vi "Control Panel.vi"(8 "error in (no error)":errorcluster, 11 "Power Supply.lvclass":refnum<class "Power Supply.lvclass">) -> (0 "error out":errorcluster, 3 "Power Supply.lvclass out":refnum<class "Power Supply.lvclass">)   [LabVIEW 2009, in "Power Supply.lvclass"]
uses:
  Power Supply.lvclass
  Utility Classes/InstrPtr/InstrPtr.lvclass
  Magnet status.ctl
  Power Supply.lvclass/Power Supply.ctl
  Global/Relative Sound Files.vi
  File IO/File IO.lvclass
panel:
  out "Was at persistent?":bool
  in  "Return to \npersistent?":bool
  out "log counter":dbl
  out "Going to Field?":bool
  out "Current Field":dbl[unit]
  out "Update UI":bool
  out "Status":T1
  out "*ips120":T2
  in  "Abort Field Sweep":bool
  out "done?":bool
  out "ILM Shut Down?":bool
  out "SH On":bool caption="Switch Heater"
  out "Persistent Mode":bool
  in  "SHcontrol":bool caption="Switch Heater"
  in  "gotopersistent":bool
  out "active":bool
  in  "Train\nMagnet":bool
  out "Busy":bool
  out "ready?":bool
  in  "rate":dbl[unit]=0.016666666666666666 caption="Rate" min=0.0 max=0.25
  in  "Goto":dbl[unit]
  in  "Clamp":bool
  in  "Check for Magnet":bool
  in  "Hold":bool
  in  "Goto Zero":bool
  in  "Goto Field":bool
  in  "endprgm":bool
  # "Magnet Control Panel"
  # "(at current field)"
  # "Off"
  # "On"
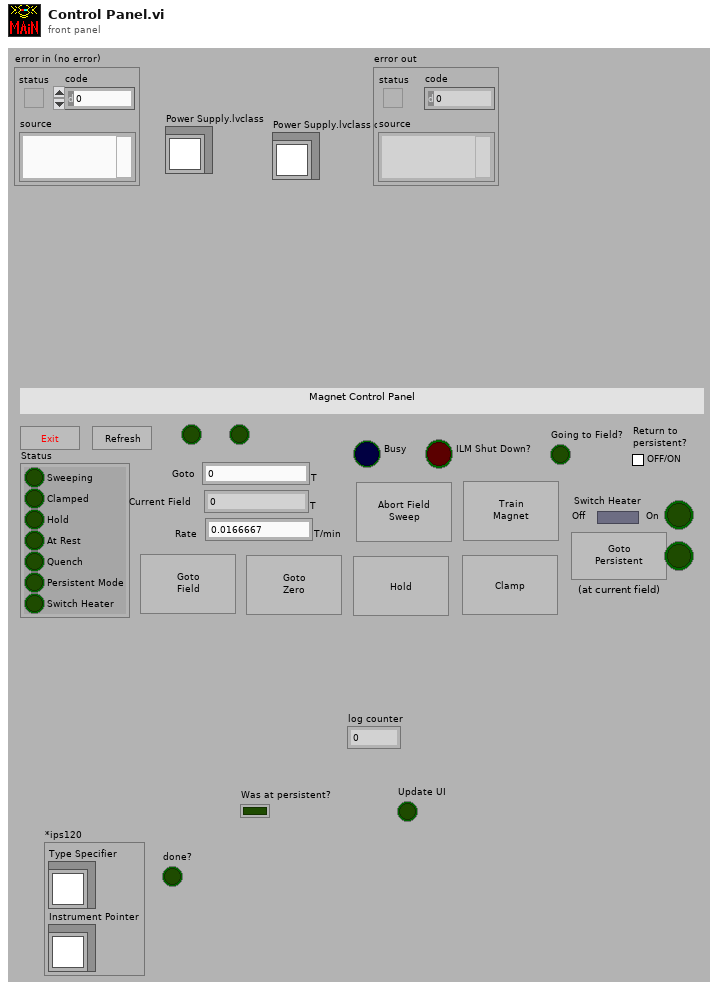
[diagram p1: front panel]
types:
  T1 = typedef "Power Supply.lvclass/Magnet status.ctl" = cluster{"Sweeping":bool, "Clamped":bool, "Hold":bool, "At Rest":bool, "Quench":bool, "Persistent Mode":bool, "Switch Heater":bool}
  T2 = cluster{"Type Specifier":refnum<class "Power Supply.lvclass">, "Instrument Pointer":refnum<class "InstrPtr.lvclass">}
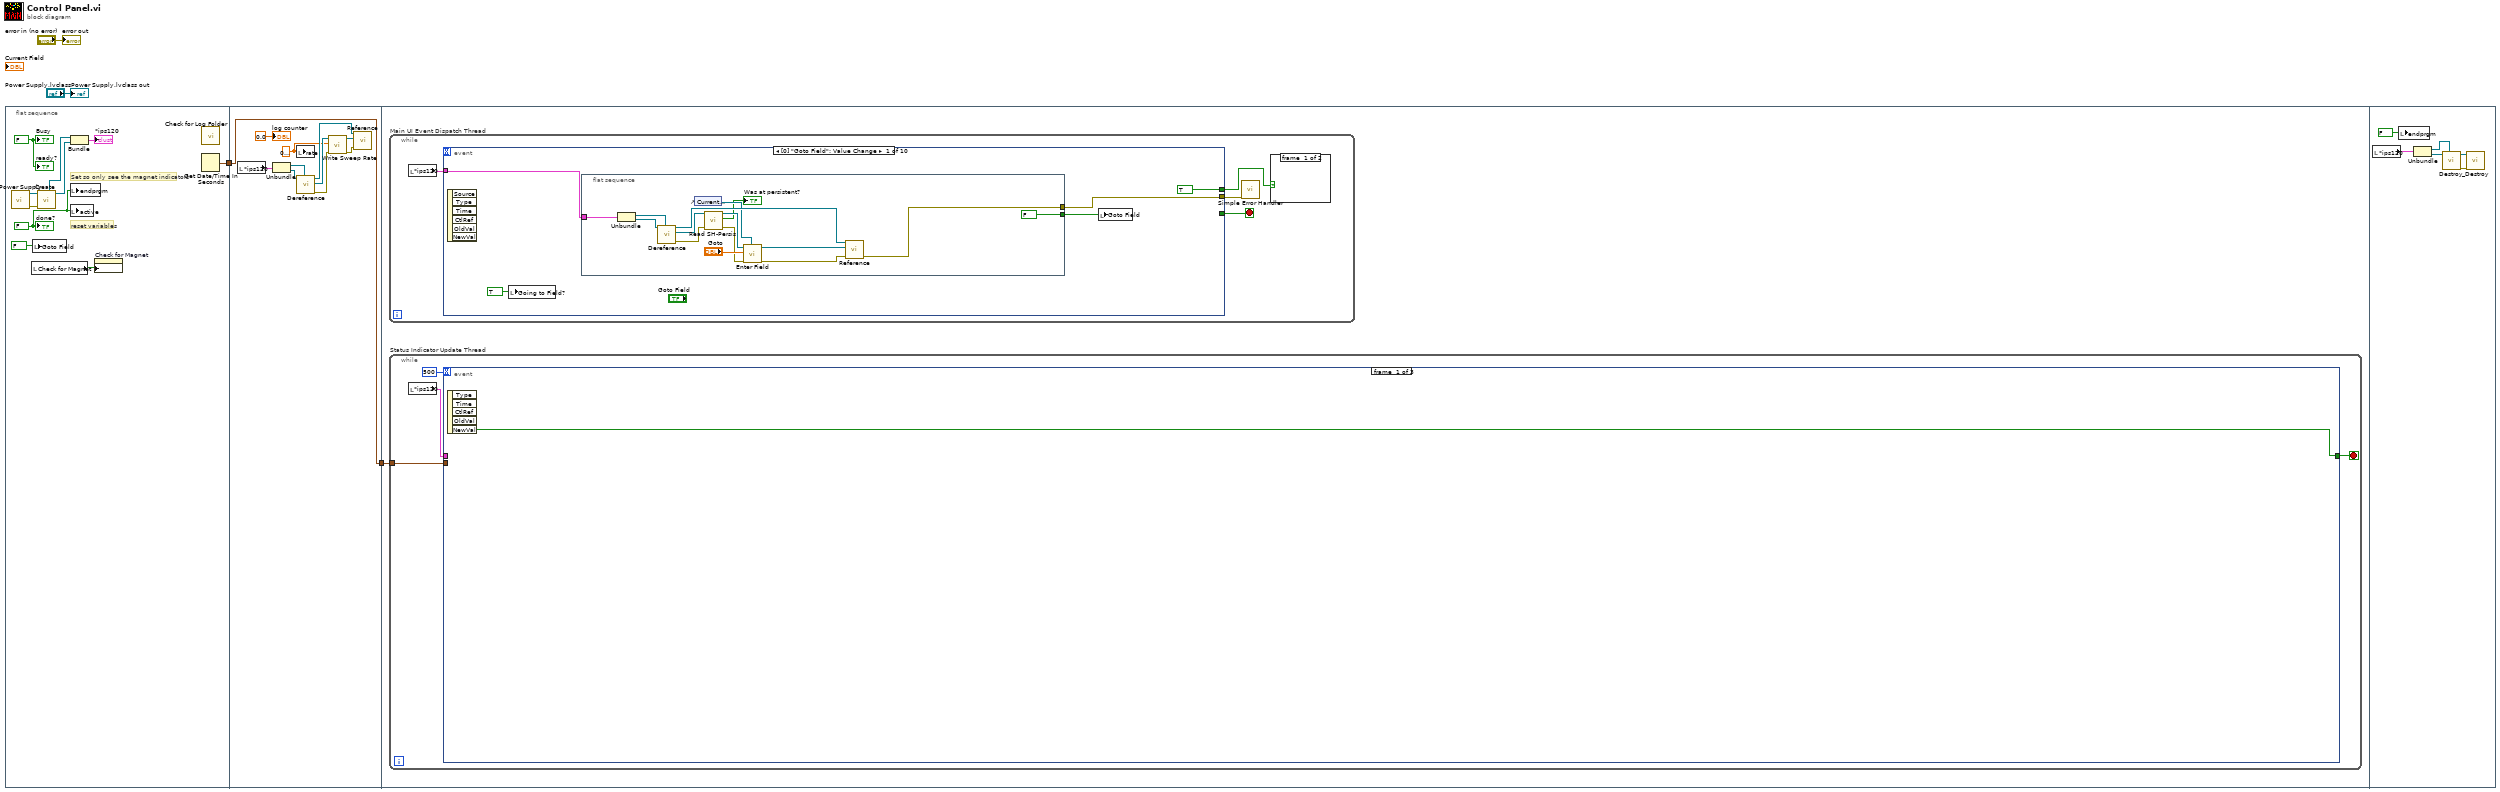
[diagram p0: block diagram]
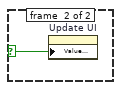
[diagram p2: hidden frame]
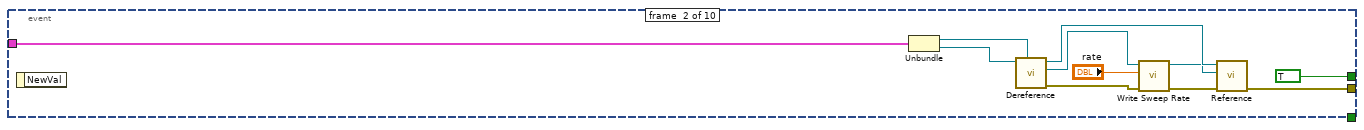
[diagram p3: hidden frame]
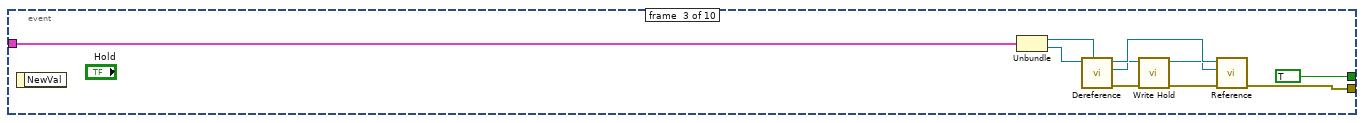
[diagram p4: hidden frame]
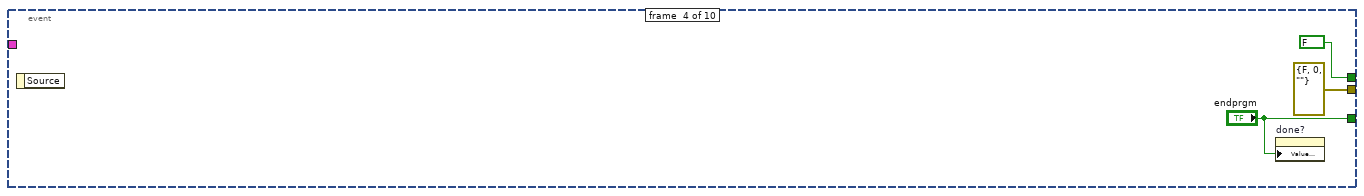
[diagram p5: hidden frame]
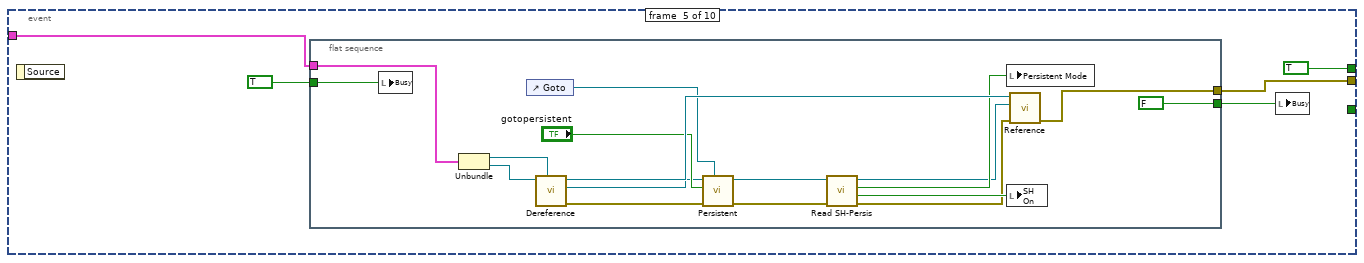
[diagram p6: hidden frame]
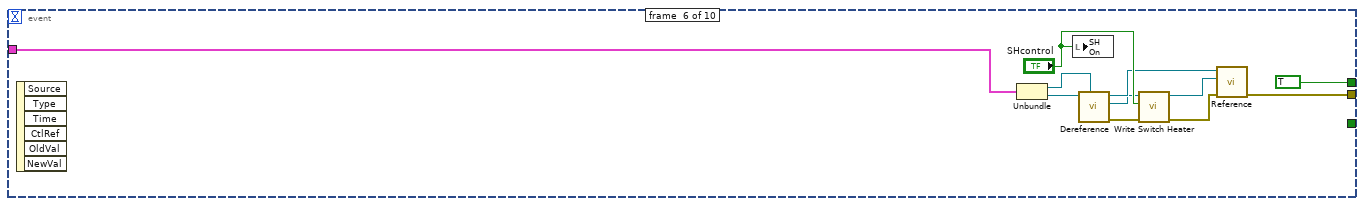
[diagram p7: hidden frame]
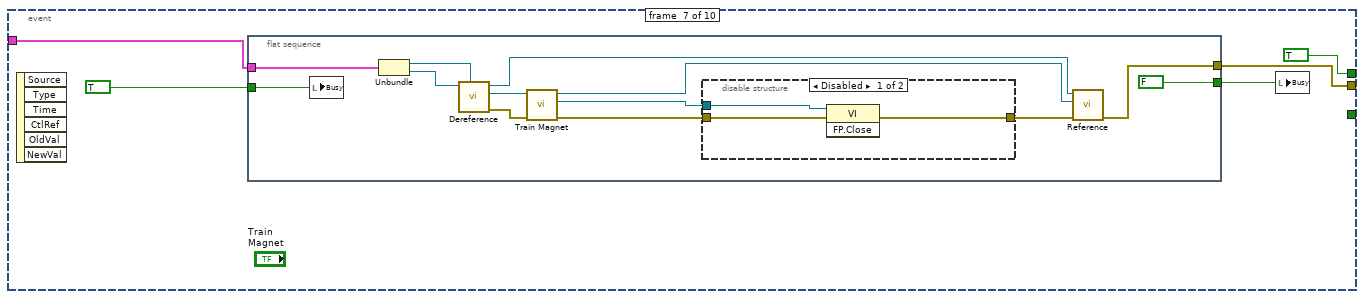
[diagram p8: hidden frame]
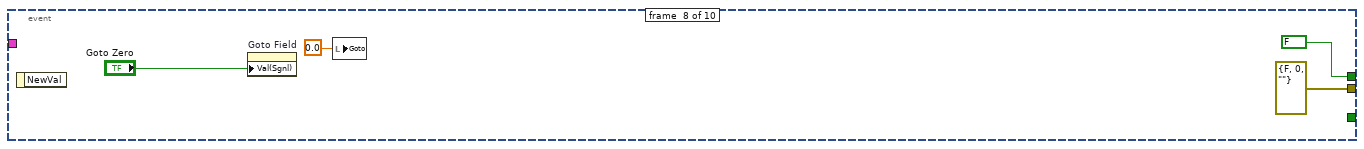
[diagram p10: hidden frame]
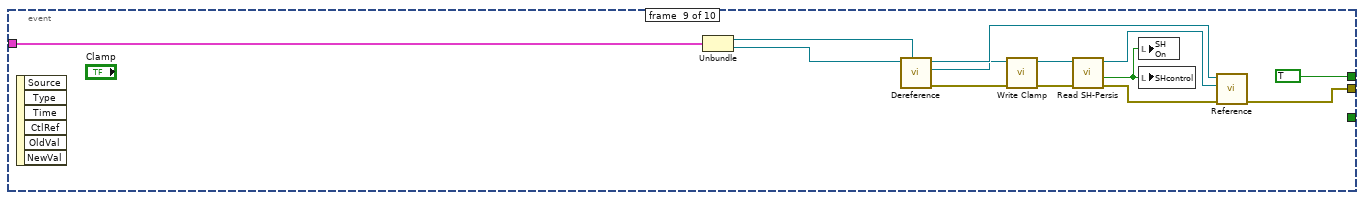
[diagram p11: hidden frame]
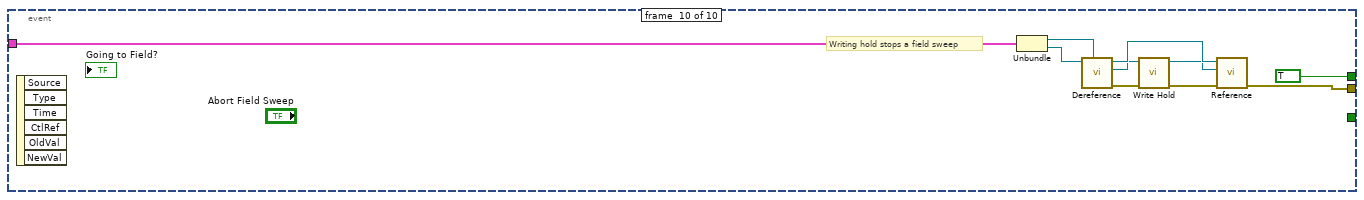
[diagram p12: hidden frame]
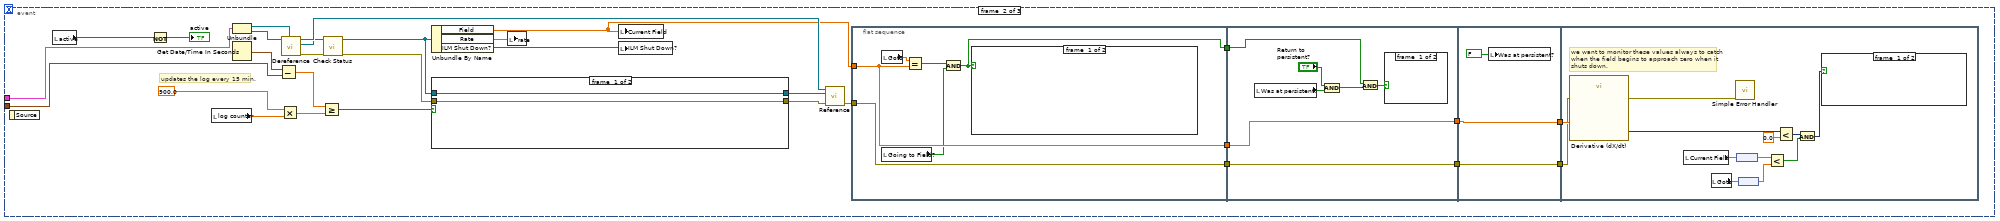
[diagram p13: hidden frame]
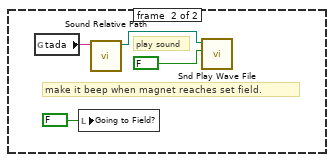
[diagram p14: hidden frame]
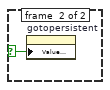
[diagram p15: hidden frame]
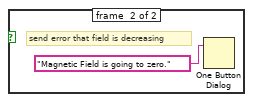
[diagram p16: hidden frame]
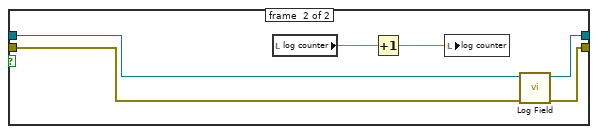
[diagram p17: hidden frame]
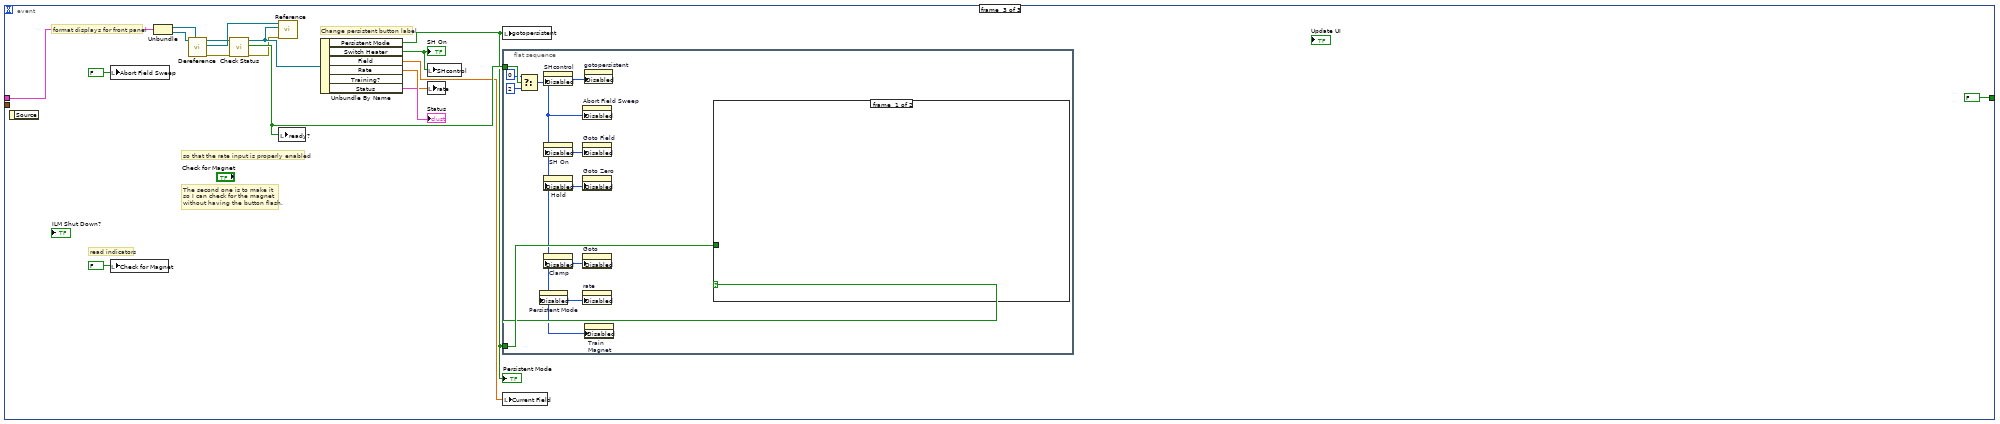
[diagram p18: hidden frame]
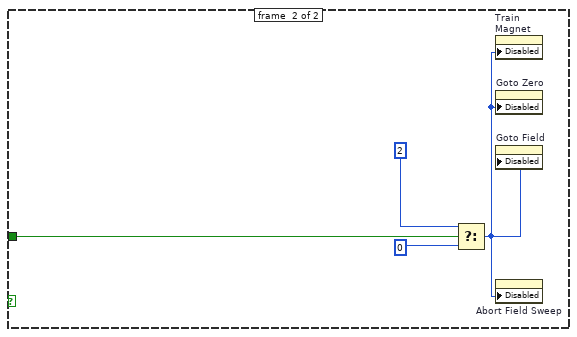
[diagram p19: hidden frame]
diagram:
  n1 = flat-sequence {
    tunnel: [w5] -> w2
    tunnel: w2 -> [w16]
    tunnel: [w16] -> w1
    tunnel: w1 -> [w26]
    frame #0 {
      w14 = FALSE
      w12 = FALSE
      # "Set so only see the magnet indicators"
      # "reset variables"
      n2 = call "Power Supply.vi"() -> ("error out"=w7:errorcluster, "Power Supply out"=w11:refnum<class "Power Supply.lvclass">)  [unwired: 10 in]
      n3 = local read "Check for Magnet"() -> (w13:bool)
      n4 = local write "Goto Field"(FALSE ("active")) -> ()
      n5 = call "Create.vi"("error in (no error)"=w7, "Instrument in"=w11) -> ("Instrument Pointer"=w10:refnum<class "InstrPtr.lvclass">, "Type Specifier"=w9:refnum<class "Power Supply.lvclass">)  [unwired: 7 in, 1 out]
      n6 = Bundle("Type Specifier"=w9, "Instrument Pointer"=w10) -> (→"*ips120":T2)  [unwired: 1 in]
      n7 = local write "endprgm"(w12) -> ()
      n8 = local write "active"(w12) -> ()
      n9 = property on="Check for Magnet" class="Bool (strict)"("Value (Signaling)"=w13) -> ()  [unwired: 2 in, 2 out]
      n10 = call "Check for Log Folder.vi"() -> ()  [unwired: 1 out]
      n11 = Get Date/Time In Seconds() -> (seconds since 1Jan1904=w5:timestamp)
      "ready?" <- w14
      "Busy" <- w14
      "done?" <- w12
    }
    frame #1 {
      w17 = dbl[unit] 0.016666666666666666 ("rate")
      n12 = local read "*ips120"() -> (w18:T2)
      n13 = Unbundle(w18) -> ("Type Specifier"=w19:refnum<class "Power Supply.lvclass">, "Instrument Pointer"=w20:refnum<class "InstrPtr.lvclass">)
      n14 = local write "rate"(w17) -> ()
      n15 = call "Dereference.vi"("Type Specifier"=w19, "InstrPtr"=w20) -> ("error out"=w24:errorcluster, "Instrument out"=w23:refnum<class "Power Supply.lvclass">, "InstrPtr out"=w21:refnum<class "InstrPtr.lvclass">)  [unwired: 7 in]
      n16 = call-dynamic "Write Sweep Rate.vi"("error in (no error)"=w24, "rate"=w17, "Power Supply in"=w23) -> ("error out"=w25:errorcluster, "Power Supply out"=w22:refnum<class "Power Supply.lvclass">)  [unwired: 7 in]
      n17 = call "Reference.vi"("error in (no error)"=w25, "Instrument"=w22, "InstrPtr in"=w21) -> ()  [unwired: 8 in, 1 out]
      "log counter" <- 0.0 ("log counter")
    }
    frame #2 {
      n18 = while "Main UI Event Dispatch Thread" {
        stop <- w29 stop-if-true
        n19 = local read "*ips120"() -> (w27:T2)
        n20 = event shown="[0] \"Goto Field\": Value Change" {
          selector: _ -> [_ _ _ _ _ _ _ _ _ _]
          dyn-events: _ -> [_ _ _ _ _ _ _ _ _ _]
          timeout: _ -> [_ _ _ _ _ _ _ _ _ _]
          tunnel: [_ _ _ "endprgm" _ _ _ _ _ _] -> w29
          tunnel: w27 -> [w36 w62 w72 _ w80 w107 w113 _ w140 w149]
          tunnel: [w34 w53 w71 errorcluster {"status"=FALSE, "code"=0, "source"=""} ("error out") w79 w101 w112 errorcluster {"status"=FALSE, "code"=0, "source"=""} ("error out") w136 w150] -> w30
          tunnel: [TRUE TRUE TRUE FALSE TRUE TRUE TRUE FALSE TRUE TRUE] -> w28
          event #0 {
            n21 = event-data() -> ()  [unwired: 7 out]
            n22 = local write "Going to Field?"(TRUE ("Going to Field?")) -> ()
            n23 = flat-sequence {
              tunnel: w36 -> [w49]
              tunnel: [FALSE ("Goto Field")] -> w35
              tunnel: [w44] -> w34
              frame #0 {
                n24 = Unbundle(w49) -> ("Type Specifier"=w51:refnum<class "Power Supply.lvclass">, "Instrument Pointer"=w50:refnum<class "InstrPtr.lvclass">)
                n25 = call "Dereference.vi"("Type Specifier"=w51, "InstrPtr"=w50) -> ("error out"=w39:errorcluster, "Instrument out"=w41:refnum<class "Power Supply.lvclass">, "InstrPtr out"=w48:refnum<class "InstrPtr.lvclass">)  [unwired: 7 in]
                n26 = control-ref of="Current Field"() -> (w43:refnum<vi>)
                n27 = call-dynamic "Read SH-Persis.vi"("error in (no error)"=w39, "Power Supply in"=w41) -> ("error out"=w38:errorcluster, "pers?"=→"Was at persistent?":bool, "Power Supply out"=w40:refnum<class "Power Supply.lvclass">)  [unwired: 4 in, 3 out]
                n28 = call-dynamic "Enter Field.vi"("Field monitor"=w43, "error in (no error)"=w38, "Target field"="Goto", "Power Supply in"=w40) -> ("error out"=w46:errorcluster, "Power Supply out"=w47:refnum<class "Power Supply.lvclass">)  [unwired: 6 in]
                n29 = call "Reference.vi"("error in (no error)"=w46, "Instrument"=w47, "InstrPtr in"=w48) -> ("error out"=w44:errorcluster)  [unwired: 8 in]
              }
            }
            n30 = local write "Goto Field"(w35) -> ()
          }
          event #1 {
            n31 = event-data() -> ()  [unwired: 2 out]
            n32 = Unbundle(w62) -> ("Type Specifier"=w61:refnum<class "Power Supply.lvclass">, "Instrument Pointer"=w60:refnum<class "InstrPtr.lvclass">)
            n33 = call "Dereference.vi"("Type Specifier"=w61, "InstrPtr"=w60) -> ("error out"=w55:errorcluster, "Instrument out"=w57:refnum<class "Power Supply.lvclass">, "InstrPtr out"=w59:refnum<class "InstrPtr.lvclass">)  [unwired: 7 in]
            n34 = call-dynamic "Write Sweep Rate.vi"("error in (no error)"=w55, "rate"="rate", "Power Supply in"=w57) -> ("error out"=w54:errorcluster, "Power Supply out"=w58:refnum<class "Power Supply.lvclass">)  [unwired: 7 in]
            n35 = call "Reference.vi"("error in (no error)"=w54, "Instrument"=w58, "InstrPtr in"=w59) -> ("error out"=w53:errorcluster)  [unwired: 8 in]
          }
          event #2 {
            n36 = event-data() -> ()  [unwired: 2 out]
            n37 = Unbundle(w72) -> ("Type Specifier"=w69:refnum<class "Power Supply.lvclass">, "Instrument Pointer"=w70:refnum<class "InstrPtr.lvclass">)
            n38 = call "Dereference.vi"("Type Specifier"=w69, "InstrPtr"=w70) -> ("error out"=w64:errorcluster, "Instrument out"=w67:refnum<class "Power Supply.lvclass">, "InstrPtr out"=w68:refnum<class "InstrPtr.lvclass">)  [unwired: 7 in]
            n39 = call-dynamic "Write Hold.vi"("error in (no error)"=w64, "Power Supply in"=w67) -> ("error out"=w65:errorcluster, "Power Supply out"=w66:refnum<class "Power Supply.lvclass">)  [unwired: 8 in]
            n40 = call "Reference.vi"("error in (no error)"=w65, "Instrument"=w66, "InstrPtr in"=w68) -> ("error out"=w71:errorcluster)  [unwired: 8 in]
          }
          event #3 {
            n41 = event-data() -> ()  [unwired: 2 out]
            n42 = property on="done?" class="Boolean (strict)"("Value (Signaling)"="endprgm") -> ()  [unwired: 2 in, 2 out]
          }
          event #4 {
            n43 = event-data() -> ()  [unwired: 2 out]
            n44 = flat-sequence {
              tunnel: w80 -> [w97]
              tunnel: [w96] -> w79
              tunnel: TRUE -> [w82]
              tunnel: [FALSE] -> w76
              frame #0 {
                n45 = local write "Busy"(w82) -> ()
                n46 = Unbundle(w97) -> ("Type Specifier"=w90:refnum<class "Power Supply.lvclass">, "Instrument Pointer"=w89:refnum<class "InstrPtr.lvclass">)
                n47 = control-ref of="Goto"() -> (w92:refnum<vi>)
                n48 = call "Dereference.vi"("Type Specifier"=w90, "InstrPtr"=w89) -> ("error out"=w87:errorcluster, "Instrument out"=w88:refnum<class "Power Supply.lvclass">, "InstrPtr out"=w93:refnum<class "InstrPtr.lvclass">)  [unwired: 7 in]
                n49 = call-dynamic "Persistent.vi"("Field monitor ref"=w92, "error in (no error)"=w87, "Go to persistent mode?"="gotopersistent", "Power Supply in"=w88) -> ("error out"=w95:errorcluster, "Power Supply out"=w94:refnum<class "Power Supply.lvclass">)  [unwired: 6 in]
                n50 = call-dynamic "Read SH-Persis.vi"("error in (no error)"=w95, "Power Supply in"=w94) -> ("error out"=w83:errorcluster, "SHon?"=w85:bool, "pers?"=w86:bool, "Power Supply out"=w84:refnum<class "Power Supply.lvclass">)  [unwired: 4 in, 2 out]
                n51 = local write "Persistent Mode"(w86) -> ()
                n52 = local write "SH On"(w85) -> ()
                n53 = call "Reference.vi"("error in (no error)"=w83, "Instrument"=w84, "InstrPtr in"=w93) -> ("error out"=w96:errorcluster)  [unwired: 8 in]
              }
            }
            n54 = local write "Busy"(w76) -> ()
          }
          event #5 {
            n55 = event-data() -> ()  [unwired: 7 out]
            n56 = Unbundle(w107) -> ("Type Specifier"=w105:refnum<class "Power Supply.lvclass">, "Instrument Pointer"=w106:refnum<class "InstrPtr.lvclass">)
            n57 = local write "SH On"("SHcontrol") -> ()
            n58 = call "Dereference.vi"("Type Specifier"=w105, "InstrPtr"=w106) -> ("error out"=w100:errorcluster, "Instrument out"=w99:refnum<class "Power Supply.lvclass">, "InstrPtr out"=w104:refnum<class "InstrPtr.lvclass">)  [unwired: 7 in]
            n59 = call-dynamic "Write Switch Heater.vi"("error in (no error)"=w100, "Turn SH On?"="SHcontrol", "Power Supply in"=w99) -> ("error out"=w102:errorcluster, "Power Supply out"=w103:refnum<class "Power Supply.lvclass">)  [unwired: 7 in]
            n60 = call "Reference.vi"("error in (no error)"=w102, "Instrument"=w103, "InstrPtr in"=w104) -> ("error out"=w101:errorcluster)  [unwired: 8 in]
          }
          event #6 {
            n61 = event-data() -> ()  [unwired: 7 out]
            n62 = flat-sequence {
              tunnel: w113 -> [w126]
              tunnel: [w122] -> w112
              tunnel: [FALSE] -> w110
              tunnel: TRUE -> [w117]
              frame #0 {
                n63 = local write "Busy"(w117) -> ()
                n64 = Unbundle(w126) -> ("Type Specifier"=w125:refnum<class "Power Supply.lvclass">, "Instrument Pointer"=w124:refnum<class "InstrPtr.lvclass">)
                n65 = call "Dereference.vi"("Type Specifier"=w125, "InstrPtr"=w124) -> ("error out"=w120:errorcluster, "Instrument out"=w121:refnum<class "Power Supply.lvclass">, "InstrPtr out"=w123:refnum<class "InstrPtr.lvclass">)  [unwired: 7 in]
                n66 = call-dynamic "Train Magnet.vi"("error in (no error)"=w120, "Power Supply in"=w121) -> ("error out"=w115:errorcluster, "This VI"=w116:refnum<vi>, "Power Supply out"=w119:refnum<class "Power Supply.lvclass">)  [unwired: 7 in]
                n67 = disable-structure shown="Disabled" {
                  disable-tunnel: w116 -> [w129 _]
                  disable-tunnel: w115 -> [w128 w130]
                  disable-tunnel: [w127 w130] -> w114
                  frame #0 {
                    n68 = invoke class="VI" method="FP.Close"(reference=w129, error in=w128) -> (error out=w127:errorcluster)  [unwired: 1 in, 2 out]
                  }
                  frame #1 {
                  }
                }
                n69 = call "Reference.vi"("error in (no error)"=w114, "Instrument"=w119, "InstrPtr in"=w123) -> ("error out"=w122:errorcluster)  [unwired: 8 in]
              }
            }
            n70 = local write "Busy"(w110) -> ()
          }
          event #7 {
            n71 = event-data() -> ()  [unwired: 2 out]
            n72 = property on="Goto Field" class="Bool (strict)"("Val(Sgnl)"="Goto Zero") -> ()  [unwired: 2 in, 2 out]
            n73 = local write "Goto"(dbl[unit] 0.0 ("Goto")) -> ()
          }
          event #8 {
            n74 = event-data() -> ()  [unwired: 7 out]
            n75 = Unbundle(w140) -> ("Type Specifier"=w144:refnum<class "Power Supply.lvclass">, "Instrument Pointer"=w143:refnum<class "InstrPtr.lvclass">)
            n76 = call "Dereference.vi"("Type Specifier"=w144, "InstrPtr"=w143) -> ("error out"=w139:errorcluster, "Instrument out"=w141:refnum<class "Power Supply.lvclass">, "InstrPtr out"=w142:refnum<class "InstrPtr.lvclass">)  [unwired: 7 in]
            n77 = call-dynamic "Write Clamp.vi"("error in (no error)"=w139, "Power Supply in"=w141) -> ("error out"=w146:errorcluster, "Power Supply out"=w147:refnum<class "Power Supply.lvclass">)  [unwired: 8 in]
            n78 = call-dynamic "Read SH-Persis.vi"("error in (no error)"=w146, "Power Supply in"=w147) -> ("error out"=w138:errorcluster, "SHon?"=w145:bool, "Power Supply out"=w137:refnum<class "Power Supply.lvclass">)  [unwired: 4 in, 3 out]
            n79 = local write "SH On"(w145) -> ()
            n80 = local write "SHcontrol"(w145) -> ()
            n81 = call "Reference.vi"("error in (no error)"=w138, "Instrument"=w137, "InstrPtr in"=w142) -> ("error out"=w136:errorcluster)  [unwired: 8 in]
          }
          event #9 {
            # "Writing hold stops a field sweep"
            n82 = event-data() -> ()  [unwired: 7 out]
            n83 = Unbundle(w149) -> ("Type Specifier"=w157:refnum<class "Power Supply.lvclass">, "Instrument Pointer"=w156:refnum<class "InstrPtr.lvclass">)
            n84 = call "Dereference.vi"("Type Specifier"=w157, "InstrPtr"=w156) -> ("error out"=w154:errorcluster, "Instrument out"=w151:refnum<class "Power Supply.lvclass">, "InstrPtr out"=w155:refnum<class "InstrPtr.lvclass">)  [unwired: 7 in]
            n85 = call-dynamic "Write Hold.vi"("error in (no error)"=w154, "Power Supply in"=w151) -> ("error out"=w153:errorcluster, "Power Supply out"=w152:refnum<class "Power Supply.lvclass">)  [unwired: 8 in]
            n86 = call "Reference.vi"("error in (no error)"=w153, "Instrument"=w152, "InstrPtr in"=w155) -> ("error out"=w150:errorcluster)  [unwired: 8 in]
          }
        }
        n87 = call <vilib>:"Simple Error Handler.vi"("error in (no error)"=w30) -> ()  [unwired: 4 in, 5 out]
        n88 = case shown="True" w28 {
          selector: w28 -> [_ w31]
          frame #0 {
          }
          frame #1 {
            n89 = property on="Update UI" class="Bool (strict)"("Value (Signaling)"=w31) -> ()  [unwired: 2 in, 2 out]
          }
        }
      }
      n90 = while "Status Indicator Update Thread" {
        tunnel: w26 -> [w158]
        stop <- w160 stop-if-true
        n91 = local read "*ips120"() -> (w159:T2)
        n92 = event shown="[1] Timeout" {
          selector: _ -> [_ _ _]
          dyn-events: _ -> [_ _ _]
          timeout: 500 -> [_ _ _]
          tunnel: [w162 _ FALSE] -> w160
          tunnel: w159 -> [_ w190 w241]
          tunnel: w158 -> [_ w189 _]
          event #0 {
            n93 = event-data() -> ("NewVal"=w162:bool)  [unwired: 5 out]
          }
          event #1 {
            # "updates the log every 15 min."
            n94 = event-data() -> ()  [unwired: 2 out]
            n95 = local read "active"() -> (w192:bool)
            n96 = Not(x=w192) -> (.not. x?=→"active":bool)
            n97 = local read "log counter"() -> (w172:dbl)
            n98 = Unbundle(w190) -> ("Type Specifier"=w185:refnum<class "Power Supply.lvclass">, "Instrument Pointer"=w186:refnum<class "InstrPtr.lvclass">)
            n99 = Get Date/Time In Seconds() -> (seconds since 1Jan1904=w175:timestamp)
            n100 = Subtract(x=w175, y=w189) -> (x-y=w170:dbl)
            n101 = Multiply(x=900.0 ("millisecond multiple"), y=w172) -> (x*y=w171:dbl)
            n102 = call "Dereference.vi"("Type Specifier"=w185, "InstrPtr"=w186) -> ("error out"=w184:errorcluster, "Instrument out"=w183:refnum<class "Power Supply.lvclass">, "InstrPtr out"=w187:refnum<class "InstrPtr.lvclass">)  [unwired: 7 in]
            n103 = Greater Or Equal?(x=w170, y=w171) -> (x >= y?=w176:bool)
            n104 = call-dynamic "Check Status.vi"("error in (no error)"=w184, "Power Supply in"=w183) -> ("error out"=w177:errorcluster, "Power Supply out"=w178:refnum<class "Power Supply.lvclass">)  [unwired: 6 in, 2 out]
            n105 = Unbundle By Name(w178) -> ("Field"=w182:dbl[unit], "Rate"=w174:dbl[unit], "ILM Shut Down?"=w188:bool)
            n106 = case shown="True" w176 {
              tunnel: [w228 w234] -> w180
              tunnel: [w227 w233] -> w179
              tunnel: w178 -> [w228 w232]
              tunnel: w177 -> [w227 w231]
              frame #0 {
              }
              frame #1 {
                n107 = local read "log counter"() -> (w230:dbl)
                n108 = Increment(x=w230) -> (x+1=w229:dbl)
                n109 = local write "log counter"(w229) -> ()
                n110 = call "Log Field.vi"("error in (no error)"=w231, "Power Supply In"=w232) -> ("error out"=w233:errorcluster, "Power Supply Out"=w234:refnum<class "Power Supply.lvclass">)  [unwired: 8 in]
              }
            }
            n111 = local write "rate"(w174) -> ()
            n112 = local write "Current Field"(w182) -> ()
            n113 = local write "ILM Shut Down?"(w188) -> ()
            n114 = call "Reference.vi"("error in (no error)"=w179, "Instrument"=w180, "InstrPtr in"=w187) -> ("error out"=w181:errorcluster)  [unwired: 8 in]
            n115 = flat-sequence {
              tunnel: w181 -> [w198]
              tunnel: w182 -> [w196]
              tunnel: [w196] -> w169
              tunnel: [w198] -> w168
              tunnel: [w193] -> w167
              tunnel: w169 -> [w209]
              tunnel: [w209] -> w166
              tunnel: w168 -> [w208]
              tunnel: [w208] -> w164
              tunnel: w167 -> [w206]
              tunnel: w166 -> [w213]
              tunnel: [w213] -> w165
              tunnel: w164 -> [w212]
              tunnel: [w212] -> w163
              tunnel: w165 -> [w225]
              tunnel: w163 -> [w224]
              frame #0 {
                n116 = local read "Goto"() -> (w197:dbl[unit])
                n117 = local read "Going to Field?"() -> (w194:bool)
                n118 = Equal?(x=w197, y=w196) -> (x = y?=w195:bool)
                n119 = And(x=w195, y=w194) -> (x .and. y?=w193:bool)
                n120 = case shown="True" w193 {
                  frame #0 {
                  }
                  frame #1 {
                    # "make it beep when magnet reaches set field."
                    # "play sound"
                    n121 = global read "Relative Sound Files.vi" "tada"() -> (w200:string)
                    n122 = local write "Going to Field?"(FALSE ("Going to Field?")) -> ()
                    n123 = call "Sound Relative Path.vi"("Sound"=w200) -> ("Relative Path"=w201:path)  [unwired: 10 in]
                    n124 = call <vilib>:"Snd Play Wave File.vi"("wait until finish (T)"=FALSE, "wave file path"=w201) -> ()  [unwired: 1 in, 9 out]
                  }
                }
              }
              frame #1 {
                n125 = local read "Was at persistent?"() -> (w205:bool)
                n126 = And(x="Return to \npersistent?", y=w205) -> (x .and. y?=w203:bool)
                n127 = And(x=w206, y=w203) -> (x .and. y?=w207:bool)
                n128 = case shown="True" w207 {
                  selector: w207 -> [_ w210]
                  frame #0 {
                  }
                  frame #1 {
                    n129 = property on="gotopersistent" class="Bool (strict)"("Value (Signaling)"=w210) -> ()  [unwired: 2 in, 2 out]
                  }
                }
              }
              frame #2 {
                n130 = local write "Was at persistent?"(FALSE ("Was at persistent?")) -> ()
              }
              frame #3 {
                # "we want to monitor these values always to catch\nwhen the field begins to approach zero when it\nshuts down."
                n131 = call "Derivative (dX/dt)"("error in (no error)"=w224, "Signals"=w225) -> ("error out"=w219:errorcluster, "Result"=w223:dynamicdata)  [unwired: 4 out]
                n132 = local read "Current Field"() -> (w215:dbl[unit])
                n133 = local read "Goto"() -> (w217:dbl[unit])
                n134 = call <vilib>:"Simple Error Handler.vi"("error in (no error)"=w219) -> ()  [unwired: 4 in, 5 out]
                n135 = node(w215) -> (w214:dbl)
                n136 = node(w217) -> (w216:dbl)
                n137 = Less?(x=w214, y=w216) -> (x < y?=w218:bool)
                n138 = Less?(x=w223, y=0.0) -> (x < y?=w221:dynamicdata)
                n139 = And(x=w221, y=w218) -> (x .and. y?=w220:dynamicdata)
                n140 = case shown="True" w220 {
                  frame #0 {
                  }
                  frame #1 {
                    # "send error that field is decreasing"
                    n141 = One Button Dialog(message="Magnetic Field is going to zero.") -> ()  [unwired: 1 in, 1 out]
                  }
                }
              }
            }
          }
          event #2 {
            # "format displays for front panel"
            # "read indicators"
            # "so that the rate input is properly enabled"
            # "Change persistent button label"
            # "The second one is to make it\nso I can check for the magnet\nwithout having the button flash."
            n142 = event-data() -> ()  [unwired: 2 out]
            n143 = local write "Abort Field Sweep"(FALSE ("Abort Field Sweep")) -> ()
            n144 = local write "Check for Magnet"(FALSE) -> ()
            n145 = Unbundle(w241) -> ("Type Specifier"=w242:refnum<class "Power Supply.lvclass">, "Instrument Pointer"=w247:refnum<class "InstrPtr.lvclass">)
            n146 = call "Dereference.vi"("Type Specifier"=w242, "InstrPtr"=w247) -> ("error out"=w246:errorcluster, "Instrument out"=w245:refnum<class "Power Supply.lvclass">, "InstrPtr out"=w243:refnum<class "InstrPtr.lvclass">)  [unwired: 7 in]
            n147 = call-dynamic "Check Status.vi"("error in (no error)"=w246, "Power Supply in"=w245) -> ("error out"=w240:errorcluster, "Ready?"=w249:bool, "Power Supply out"=w244:refnum<class "Power Supply.lvclass">)  [unwired: 6 in, 1 out]
            n148 = call "Reference.vi"("error in (no error)"=w240, "Instrument"=w244, "InstrPtr in"=w243) -> ()  [unwired: 8 in, 1 out]
            n149 = local write "ready?"(w249) -> ()
            n150 = Unbundle By Name(w244) -> ("Persistent Mode"=w237:bool, "Switch Heater"=w248:bool, "Field"=w238:dbl[unit], "Rate"=w235:dbl[unit], "Status"=→"Status":T1)  [unwired: 1 out]
            "Persistent Mode" <- w237
            "SH On" <- w248
            n151 = local write "SHcontrol"(w248) -> ()
            n152 = local write "rate"(w235) -> ()
            n153 = local write "gotopersistent"(w237) -> ()
            n154 = flat-sequence {
              tunnel: w237 -> [w256]
              tunnel: w249 -> [w255]
              frame #0 {
                n155 = Select(t=0, s=w255, f=2) -> (s? t:f=w252:i32)
                n156 = property on="Persistent Mode" class="Boolean (strict)"("Disabled"=w252) -> ()  [unwired: 2 in, 2 out]
                n157 = property on="SHcontrol" class="Boolean (strict)"("Disabled"=w252) -> ()  [unwired: 2 in, 2 out]
                n158 = property on="SH On" class="Boolean (strict)"("Disabled"=w252) -> ()  [unwired: 2 in, 2 out]
                n159 = property on="Hold" class="Boolean"("Disabled"=w252) -> ()  [unwired: 2 in, 2 out]
                n160 = property on="Clamp" class="Boolean"("Disabled"=w252) -> ()  [unwired: 2 in, 2 out]
                n161 = property on="Abort Field Sweep" class="Bool (strict)"("Disabled"=w252) -> ()  [unwired: 2 in, 2 out]
                n162 = property on="Goto Field" class="Bool (strict)"("Disabled"=w252) -> ()  [unwired: 2 in, 2 out]
                n163 = property on="Goto Zero" class="Bool"("Disabled"=w252) -> ()  [unwired: 2 in, 2 out]
                n164 = property on="Goto" class="DigNum (strict)"("Disabled"=w252) -> ()  [unwired: 2 in, 2 out]
                n165 = property on="rate" class="DigNum (strict)"("Disabled"=w252) -> ()  [unwired: 2 in, 2 out]
                n166 = property on="gotopersistent" class="Bool (strict)"("Disabled"=w252) -> ()  [unwired: 2 in, 2 out]
                n167 = property on="Train\nMagnet" class="Boolean"("Disabled"=w252) -> ()  [unwired: 2 in, 2 out]
                n168 = case shown="True" w255 {
                  tunnel: w256 -> [_ w258]
                  frame #0 {
                  }
                  frame #1 {
                    n169 = Select(t=2, s=w258, f=0) -> (s? t:f=w257:i32)
                    n170 = property on="Train\nMagnet" class="Boolean"("Disabled"=w257) -> ()  [unwired: 2 in, 2 out]
                    n171 = property on="Goto Zero" class="Bool"("Disabled"=w257) -> ()  [unwired: 2 in, 2 out]
                    n172 = property on="Goto Field" class="Bool (strict)"("Disabled"=w257) -> ()  [unwired: 2 in, 2 out]
                    n173 = property on="Abort Field Sweep" class="Bool (strict)"("Disabled"=w257) -> ()  [unwired: 2 in, 2 out]
                  }
                }
              }
            }
            n174 = local write "Current Field"(w238) -> ()
          }
        }
      }
    }
    frame #3 {
      n175 = local read "*ips120"() -> (w265:T2)
      n176 = local write "endprgm"(FALSE) -> ()
      n177 = Unbundle(w265) -> ("Type Specifier"=w262:refnum<class "Power Supply.lvclass">, "Instrument Pointer"=w264:refnum<class "InstrPtr.lvclass">)
      n178 = call "Destroy.vi"("Type Specifier"=w262, "InstrPtr in"=w264) -> ("error out"=w261:errorcluster, "final Instrument"=w263:refnum<class "Power Supply.lvclass">)  [unwired: 8 in]
      n179 = call-dynamic "_Destroy.vi"("error in (no error)"=w261, "Instrument in"=w263) -> ()  [unwired: 9 in, 1 out]
    }
  }
  "Power Supply.lvclass out" <- "Power Supply.lvclass"
  "error out" <- "error in (no error)"
